vi "Station_Meteo_Miguel_Soares.vi"() -> ()   [LabVIEW 2018]
uses:
  Array station.vi
  <vilib>/Instr/_visa.llb/VISA Configure Serial Port (Instr).vi
  <vilib>/Utility/file.llb/Write Delimited Spreadsheet (string).vi
panel:
  out "String":string
  in  "Pause":bool
  in  "Sauver":bool
  in  "file path (use dialog)":path
  in  "Combo Box":string(combo)
  out "Humidité MAX":dbl
  out "Humidité MIN":dbl
  out "Témperature MAX":dbl
  out "Témperature MIN":dbl
  out "Préssion MAX":dbl
  out "Préssion MIN":dbl
  out "Préssion moyenne":dbl format="%#_4g"
  out "Humidité moyenne":dbl format="%#_4g"
  out "Waveform Graph 3":dbl[](graph)
  out "Waveform Graph 2":dbl[](graph)
  out "Waveform Graph":dbl[](graph)
  out "Température moyenne":dbl format="%#_4g"
  out "Humidité":string
  out "Presion":string
  out "Température":string
  in  "stop":bool
  in  "Nom de ressource VISA":refnum<visa-resource-name>
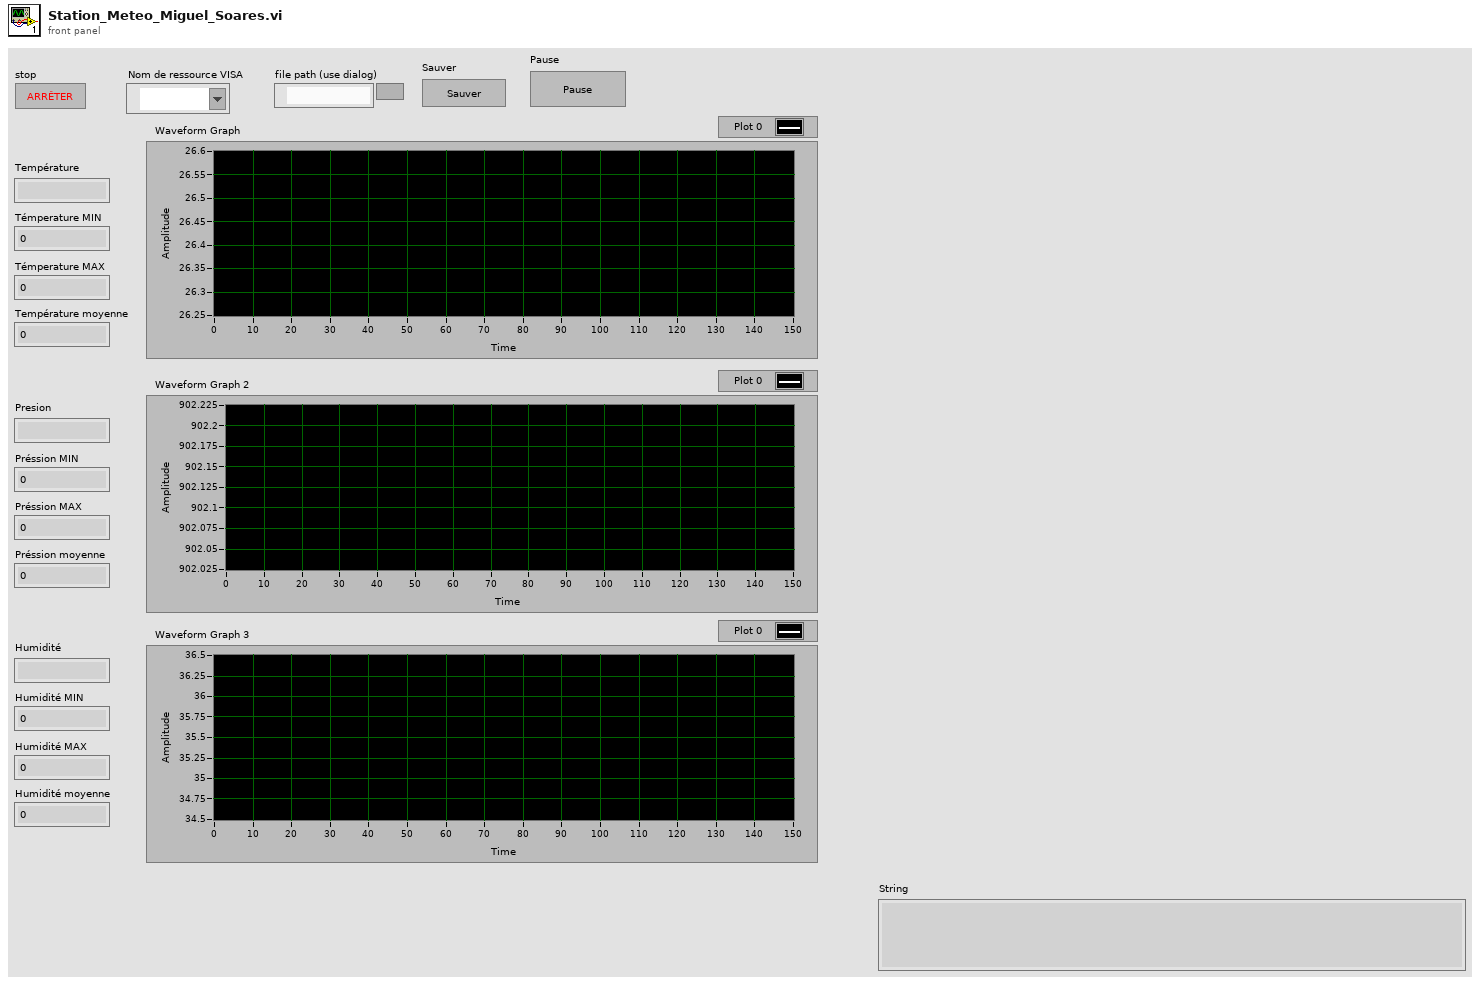
[diagram p1: front panel]
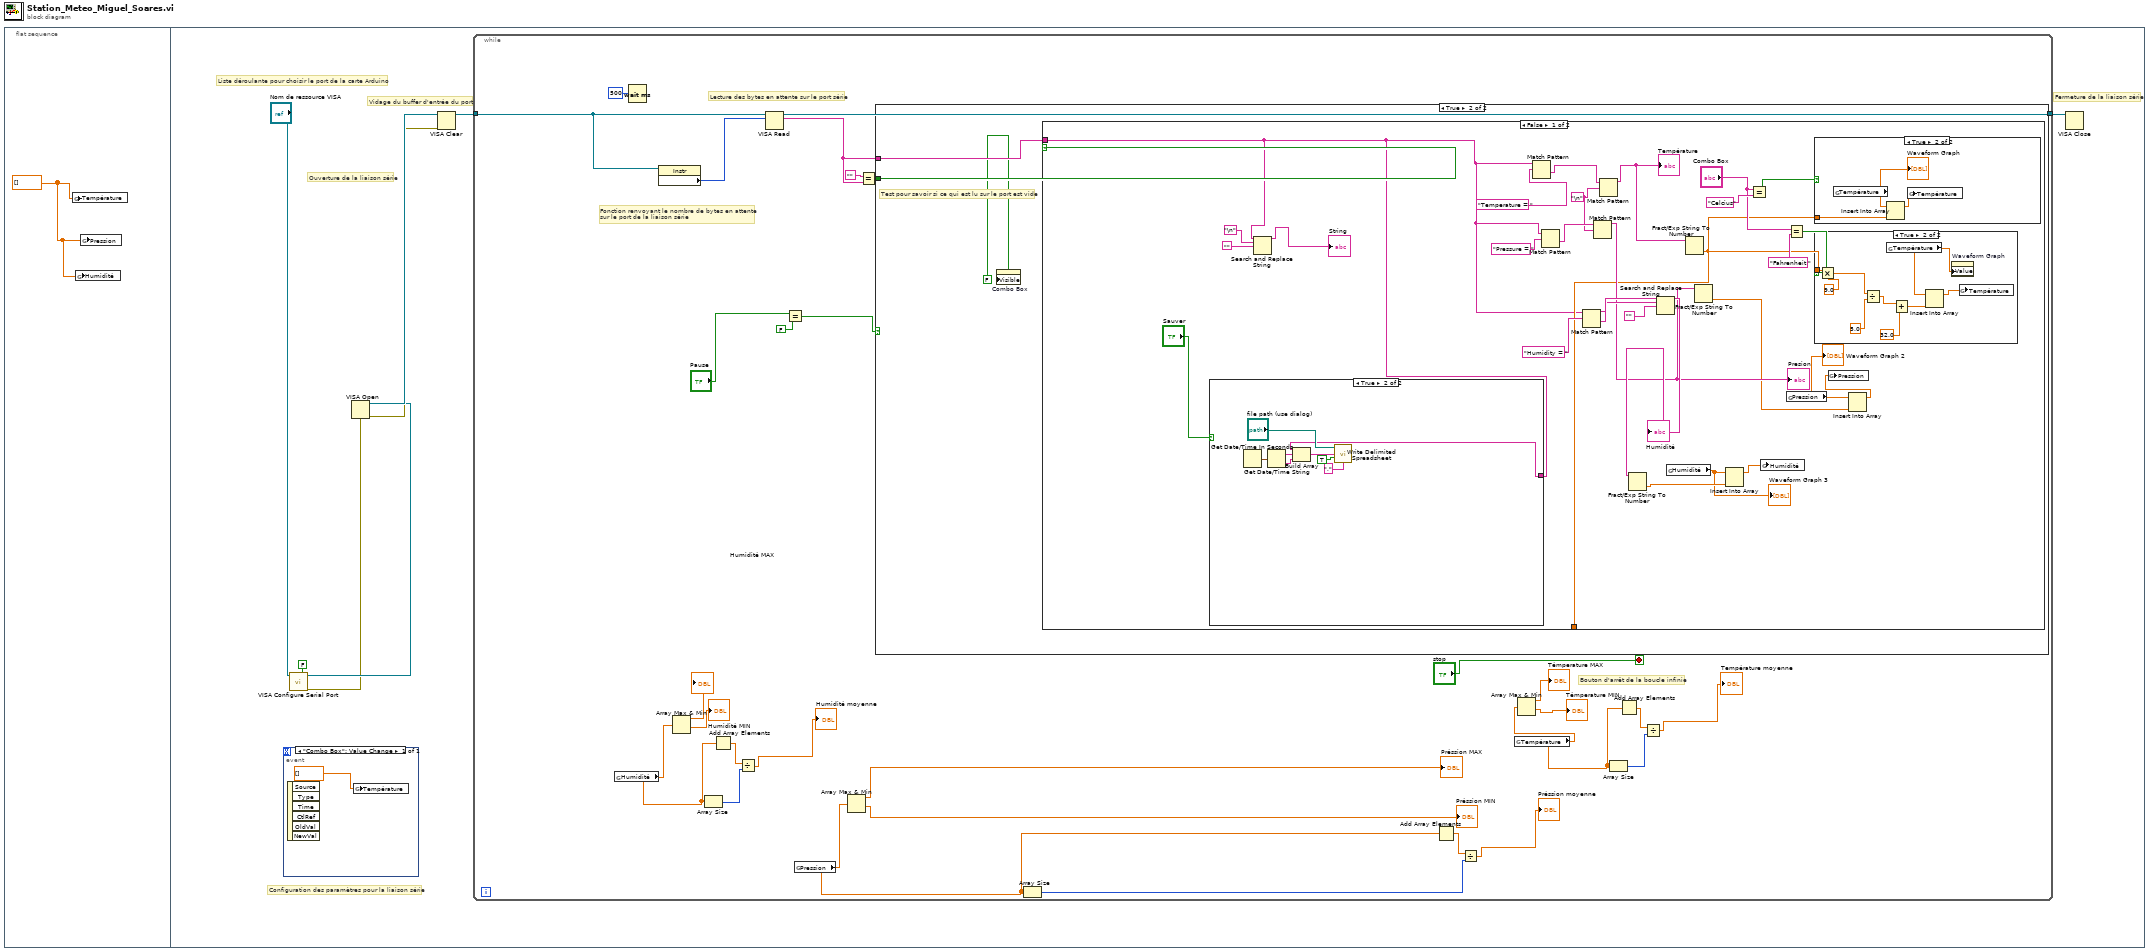
[diagram p0: block diagram]
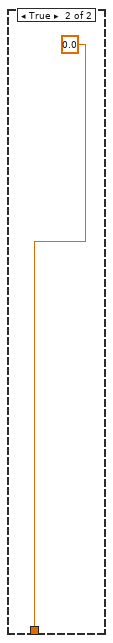
[diagram p6: hidden frame]
diagram:
  n1 = flat-sequence {
    frame #0 {
      w1 = dbl[] []
      n2 = global write "Array station.vi" "Température"(w1) -> ()
      n3 = global write "Array station.vi" "Humidité"(w1) -> ()
      n4 = global write "Array station.vi" "Pression"(w1) -> ()
    }
    frame #1 {
      # "Vidage du buffer d'entrée du port"
      # "Ouverture de la liaison série"
      # "Configuration des paramètres pour la liaison série"
      # "Liste déroulante pour choisir le port de la carte Arduino"
      # "Fermeture de la liaison série"
      n5 = event shown="[0] \"Combo Box\": Value Change" {
        selector: _ -> [_]
        dyn-events: _ -> [_]
        timeout: _ -> [_]
        event "Combo Box": Value Change {
          n6 = event-data() -> ()  [unwired: 1 in, 6 out]
          n7 = global write "Array station.vi" "Température"(dbl[] []) -> ()
        }
      }
      n8 = call-poly "VISA Configure Serial Port"("VISA resource name"="Nom de ressource VISA", "Enable Termination\nChar (T)"=FALSE ("Enable Termination\nChar (T)")) -> ("VISA resource name out"=w6:refnum<visa-resource-name>, "error out"=w4:errorcluster)  [unwired: 12 in]
      n9 = VISA Open(error in (no error)=w4, VISA resource name=w6) -> (VISA resource name=w8:refnum<visa-resource-name>, error out=w3:errorcluster)  [unwired: 3 in]
      n10 = VISA Clear(VISA resource name=w8, error in (no error)=w3) -> (VISA resource name out=w7:refnum<visa-resource-name>)  [unwired: 1 out]
      n11 = while {
        tunnel: w7 -> [w39]
        tunnel: [w37] -> w2
        stop <- "stop" stop-if-true
        # "Lecture des bytes en attente sur le port série"
        # "Fonction renvoyant le nombre de bytes en attente\nsur le port de la liaison série"
        # "Bouton d'arrêt de la boucle infinie"
        n12 = global read "Array station.vi" "Humidité"() -> (w18:dbl[])
        n13 = Wait (ms)(milliseconds to wait=u32 500 ("attente (ms)")) -> ()  [unwired: 1 out]
        n14 = property class="Instr"(reference=w39) -> ("Serial Settings:Number of Bytes at Serial Port"=w38:u32)  [unwired: 1 in, 2 out]
        n15 = Array Max & Min(array=w18) -> (max value=→"Humidité MAX":dbl, min value=→"Humidité MIN":dbl)  [unwired: 2 out]
        n16 = Array Size(array=w18) -> (size(s)=w28:i32)
        n17 = Add Array Elements(numeric array=w18) -> (sum=w29:dbl)
        n18 = Divide(x=w29, y=w28) -> (x/y=→"Humidité moyenne":dbl)
        n19 = VISA Read(VISA resource name=w39, byte count=w38) -> (VISA resource name out=w37:refnum<visa-resource-name>, read buffer=w33:string)  [unwired: 1 in, 2 out]
        n20 = Equal?(x="Pause", y=FALSE) -> (x = y?=w12:bool)
        n21 = global read "Array station.vi" "Pression"() -> (w23:dbl[])
        n22 = Array Max & Min(array=w23) -> (max value=→"Préssion MAX":dbl, min value=→"Préssion MIN":dbl)  [unwired: 2 out]
        n23 = Equal?(x="", y=w33) -> (x = y?=w34:bool)
        n24 = case shown="True" w12 {
          tunnel: w34 -> [_ w42]
          tunnel: w33 -> [_ w41]
          frame False {
          }
          frame True {
            # "Test pour savoir si ce qui est lu sur le port est vide"
            n25 = property on="Combo Box" class="CmbBox"("Visible"=FALSE) -> ()  [unwired: 2 in, 2 out]
            n26 = case shown="False" w42 {
              tunnel: w41 -> [w46 _]
              tunnel: [w48 0.0] -> _
              frame False {
                w63 = "\n"
                n27 = case shown="True" "Sauver" {
                  tunnel: w46 -> [_ w75]
                  frame False {
                  }
                  frame True {
                    n28 = Get Date/Time In Seconds() -> (seconds since 1Jan1904=w79:timestamp)
                    n29 = Get Date/Time String(seconds (now)=w79) -> (date string=w76:string, time string=w77:string)  [unwired: 2 in]
                    n30 = Build Array(w75, w76, w77) -> (w74:string[])
                    n31 = call-poly <vilib>:"Write Delimited Spreadsheet.vi"("file path (dialog if empty)"="file path (use dialog)", "1D data"=w74, "append to file? (new file:F)"=TRUE, "delimiter (\\t)"="," ("delimiter (\\t)")) -> ()  [unwired: 10 in, 2 out]
                  }
                }
                n32 = Search and Replace String(input string=w46, search string="\n", replace string="") -> (result string=→"String":string)  [unwired: 5 in, 3 out]
                n33 = Match Pattern(string=w46, regular expression="Temperature = ") -> (after substring=w66:string)  [unwired: 1 in, 3 out]
                n34 = Match Pattern(string=w46, regular expression="Pressure = ") -> (after substring=w64:string)  [unwired: 1 in, 3 out]
                n35 = Match Pattern(string=w46, regular expression="Humidity = ") -> (before substring=w70:string, after substring=w71:string)  [unwired: 1 in, 2 out]
                n36 = Match Pattern(string=w64, regular expression=w63) -> (before substring=w61:string)  [unwired: 1 in, 3 out]
                "Presion" <- w61
                n37 = Match Pattern(string=w66, regular expression=w63) -> (before substring=w60:string)  [unwired: 1 in, 3 out]
                "Température" <- w60
                n38 = Search and Replace String(input string=w71, search string=w70, replace string="") -> (result string=w62:string)  [unwired: 5 in, 3 out]
                "Humidité" <- w62
                n39 = Fract/Exp String To Number(string=w62) -> (number=w59:dbl)  [unwired: 3 in, 1 out]
                n40 = global read "Array station.vi" "Humidité"() -> (w55:dbl[])
                "Waveform Graph 3" <- w55
                n41 = Fract/Exp String To Number(string=w60) -> (number=w48:dbl)  [unwired: 3 in, 1 out]
                n42 = Fract/Exp String To Number(string=w61) -> (number=w58:dbl)  [unwired: 3 in, 1 out]
                n43 = Insert Into Array(array=w55, new element=w59) -> (w57:dbl[])  [unwired: 1 in]
                n44 = Equal?(x="Combo Box", y="Celcius") -> (x = y?=w52:bool)
                n45 = global write "Array station.vi" "Humidité"(w57) -> ()
                n46 = global read "Array station.vi" "Pression"() -> (w54:dbl[])
                "Waveform Graph 2" <- w54
                n47 = Equal?(x="Combo Box", y="Fahrenheit ") -> (x = y?=w49:bool)
                n48 = case shown="True" w52 {
                  tunnel: w48 -> [_ w89]
                  frame False {
                  }
                  frame True {
                    n49 = global read "Array station.vi" "Température"() -> (w91:dbl[])
                    "Waveform Graph" <- w91
                    n50 = Insert Into Array(array=w91, new element=w89) -> (w90:dbl[])  [unwired: 1 in]
                    n51 = global write "Array station.vi" "Température"(w90) -> ()
                  }
                }
                n52 = case shown="True" w49 {
                  tunnel: w48 -> [_ w81]
                  frame False {
                  }
                  frame True {
                    n53 = Multiply(x=w81, y=9.0) -> (x*y=w87:dbl)
                    n54 = Divide(x=w87, y=5.0) -> (x/y=w86:dbl)
                    n55 = global read "Array station.vi" "Température"() -> (w80:dbl[])
                    n56 = Add(x=w86, y=32.0) -> (x+y=w85:dbl)
                    n57 = Insert Into Array(array=w80, new element=w85) -> (w88:dbl[])  [unwired: 1 in]
                    n58 = property on="Waveform Graph" class="WFGraph (strict)"("Value"=w80) -> ()  [unwired: 2 in, 2 out]
                    n59 = global write "Array station.vi" "Température"(w88) -> ()
                  }
                }
                n60 = Insert Into Array(array=w54, new element=w58) -> (w56:dbl[])  [unwired: 1 in]
                n61 = global write "Array station.vi" "Pression"(w56) -> ()
              }
              frame True {
              }
            }
          }
        }
        n62 = Array Size(array=w23) -> (size(s)=w25:i32)
        n63 = Add Array Elements(numeric array=w23) -> (sum=w26:dbl)
        n64 = Divide(x=w26, y=w25) -> (x/y=→"Préssion moyenne":dbl)
        n65 = global read "Array station.vi" "Température"() -> (w17:dbl[])
        n66 = Array Max & Min(array=w17) -> (max value=→"Témperature MAX":dbl, min value=→"Témperature MIN":dbl)  [unwired: 2 out]
        n67 = Array Size(array=w17) -> (size(s)=w31:i32)
        n68 = Add Array Elements(numeric array=w17) -> (sum=w32:dbl)
        n69 = Divide(x=w32, y=w31) -> (x/y=→"Température moyenne":dbl)
      }
      n70 = VISA Close(VISA resource name=w2) -> ()  [unwired: 1 in, 1 out]
    }
  }
